vi "String - Add BOM if IsUnicode.vi"(5 "target length (65535)":i32=65535, 7 "Input is Unicode (varbinary)?":bool, 11 "String IN":string) -> (3 "BOM Added":string)   [LabVIEW 2020]
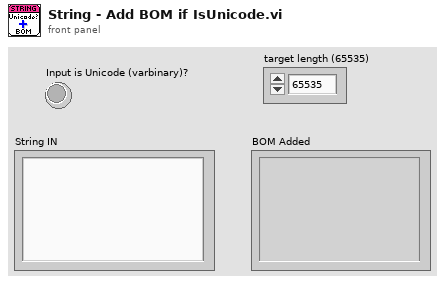
[diagram p1: front panel]
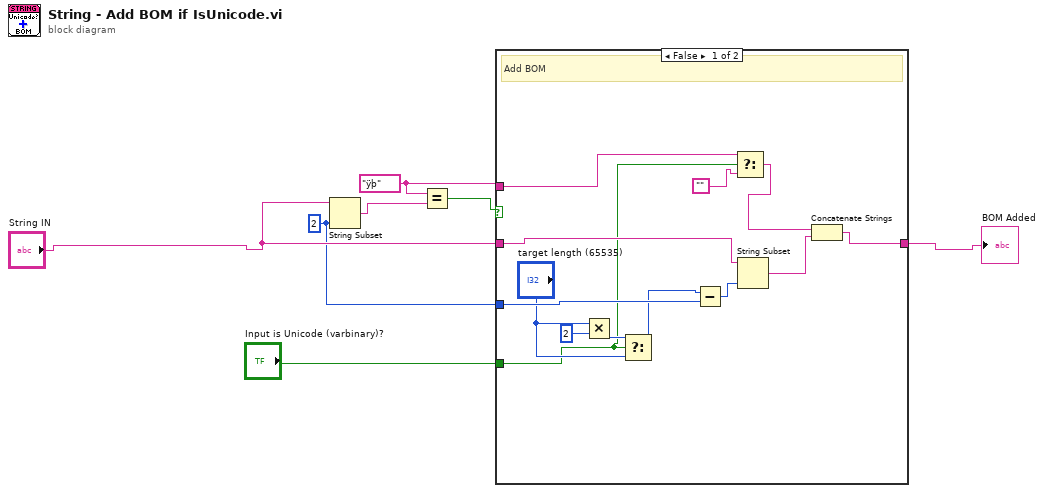
[diagram p0: block diagram]
diagram:
  w3 = "ÿþ" ("y")
  w2 = 2 ("length (rest)")
  n1 = String Subset(string="String IN", length (rest)=w2) -> (substring=w5:string)  [unwired: 1 in]
  n2 = Equal?(x=w3, y=w5) -> (x = y?=w4:bool)
  n3 = case shown="False" w4 {
    tunnel: "String IN" -> [w19 w21]
    tunnel: [w20 w21] -> w6
    tunnel: w3 -> [w10 _]
    tunnel: w2 -> [w17 _]
    tunnel: "Input is Unicode (varbinary)?" -> [w11 _]
    frame False {
      # "Add BOM"
      n4 = Multiply(x="target length (65535)", y=2) -> (x*y=w13:i32)
      n5 = Select(t=w13, s=w11, f="target length (65535)") -> (s? t:f=w15:i32)
      n6 = Subtract(x=w15, y=w17) -> (x-y=w16:i32)
      n7 = Select(t=w10, s=w11, f="") -> (s? t:f=w9:string)
      n8 = String Subset(string=w19, length (rest)=w16) -> (substring=w18:string)  [unwired: 1 in]
      n9 = Concatenate Strings(w9, w18) -> (w20:string)
    }
    frame True {
      # "Already there, no need to add"
    }
  }
  "BOM Added" <- w6
